vi "Send Receive.vi"(0 "Arduino Resource":T1={"VISA resource"="", "Board Type"=enum."Uno", "Connection Type"=enum."USB / Serial", "Bytes Per Packet (15)"=15}, 1 "Max Retries  (10)":i32=10, 5 "Data":u8[](array[numeric]), 7 "Bytes To Read (0)":u8, 9 "Time Out (100 ms)":i32=100, 11 "error in":errorcluster) -> (4 "Arduino Resource":T1={"VISA resource"="", "Board Type"=enum."Uno", "Connection Type"=enum."USB / Serial", "Bytes Per Packet (15)"=15}, 8 "Read Buffer":string, 15 "error out":errorcluster)   [LabVIEW 2015, in "LabVIEW Interface for Arduino.lvlib"]
uses:
  <vilib>/LabVIEW Interface for Arduino/LabVIEW Interface for Arduino.lvlib
  <vilib>/LabVIEW Interface for Arduino/Type Defs/Arduino Resource.ctl
  <vilib>/LabVIEW Interface for Arduino/Type Defs/Board Type.ctl
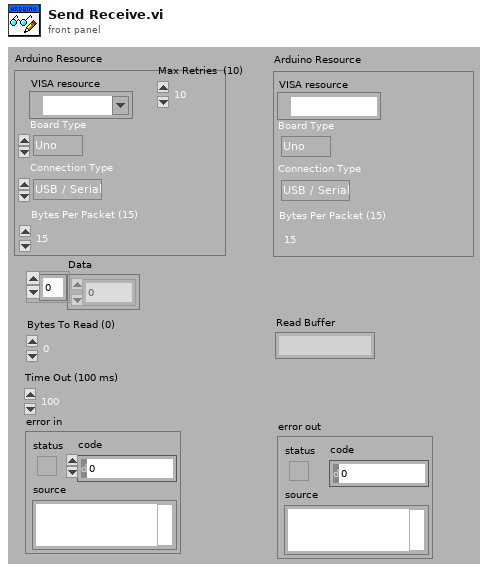
[diagram p1: front panel]
types:
  T1 = typedef "LabVIEW Interface for Arduino.lvlib/Arduino Resource.ctl" = cluster{"VISA resource":refnum<visa-resource-name>, "Board Type":T2, "Connection Type":enum8{"USB / Serial"}, "Bytes Per Packet (15)":u8}
  T2 = typedef "LabVIEW Interface for Arduino.lvlib/Board Type.ctl" = enum16{"Uno", "Dimuelanove w/Atmega 328", "Mega 2560"}
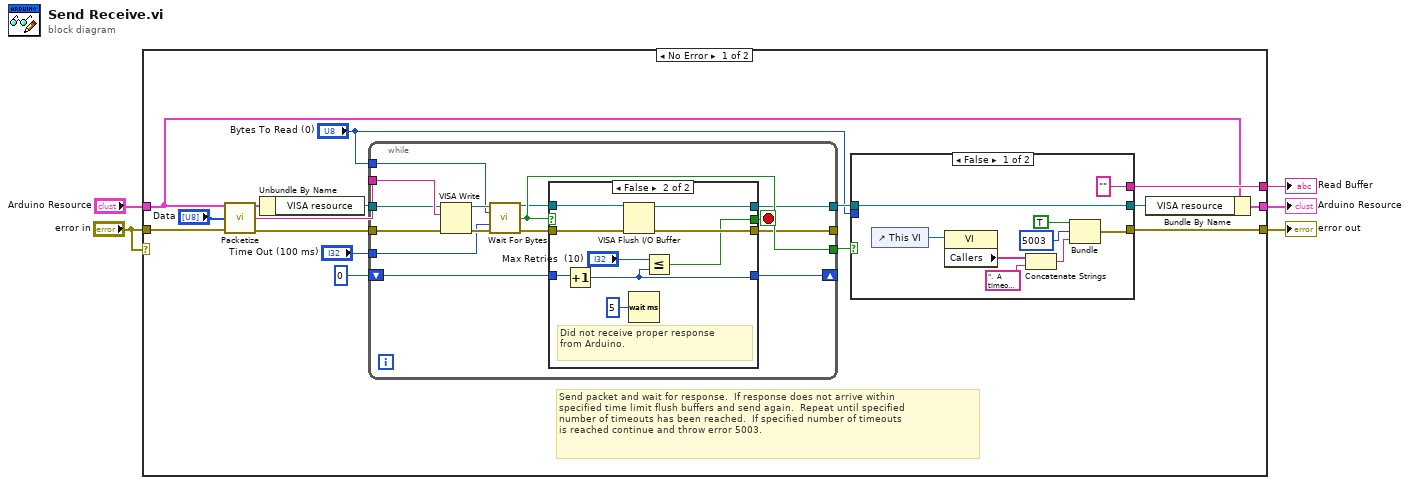
[diagram p0: block diagram]
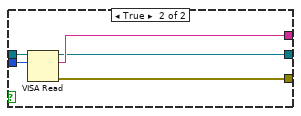
[diagram p3: hidden frame]
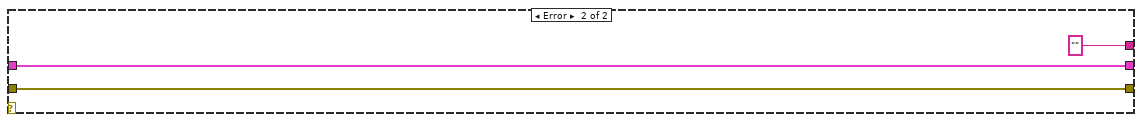
[diagram p4: hidden frame]
diagram:
  n1 = case shown="No Error" "error in" {
    tunnel: [w21 w65] -> w5
    tunnel: [w18 "" ("read buffer")] -> w4
    tunnel: "error in" -> [w6 w65]
    tunnel: "Arduino Resource" -> [w8 w66]
    tunnel: [w14 w66] -> w2
    frame No Error {
      # "Send packet and wait for response.  If response does not arrive within \nspecified time limit flush buffers and send again.  Repeat until specified \nnumber of timeouts has been reached.  If specified number of timeouts\nis reached continue and throw error 5003."
      n2 = call <vilib>:"Packetize.vi"("Arduino Resource"=w8, "Data"="Data", "error in"=w6) -> ("Arduino Resource"=w9:T1, "Packet"=w19:string, "error out"=w7:errorcluster)  [unwired: 10 in]
      n3 = Unbundle By Name(w9) -> ("VISA resource"=w16:refnum<visa-resource-name>)
      n4 = while {
        tunnel: w19 -> [w36]
        tunnel: [w24] -> w17
        tunnel: w7 -> [w33]
        tunnel: w16 -> [w32]
        tunnel: "Bytes To Read (0)" -> [w31]
        tunnel: "Time Out (100 ms)" -> [w30]
        tunnel: [w26] -> w11
        shift-right: [w28] -> _
        shift-left: 0 -> [w29]
        tunnel: [w22] -> _
        stop <- w27 stop-if-true
        n5 = VISA Write(VISA resource name=w32, write buffer=w36, error in (no error)=w33) -> (VISA resource name out=w34:refnum<visa-resource-name>, error out=w35:errorcluster)  [unwired: 1 out]
        n6 = call <vilib>:"Wait For Bytes.vi"("VISA resource"=w34, "Bytes To Read"=w31, "Time Out (100 ms)"=w30, "error in"=w35) -> ("VISA resource"=w23:refnum<visa-resource-name>, "Bytes Available?"=w26:bool, "error out"=w25:errorcluster)  [unwired: 9 in]
        n7 = case shown="False" w26 {
          selector: w26 -> [w39 _]
          tunnel: w29 -> [w40 w49]
          tunnel: [w40 w42] -> w28
          tunnel: [w39 w41] -> w27
          tunnel: w25 -> [w37 w47]
          tunnel: [w38 w46] -> w24
          tunnel: w23 -> [w38 w45]
          tunnel: [w37 w44] -> w22
          frame True {
          }
          frame False {
            # "Did not receive proper response\nfrom Arduino."
            n8 = Increment(x=w49) -> (x+1=w42:i32)
            n9 = VISA Flush I/O Buffer(VISA resource name=w45, error in (no error)=w47) -> (VISA resource name out=w46:refnum<visa-resource-name>, error out=w44:errorcluster)  [unwired: 1 in]
            n10 = Wait (ms)(milliseconds to wait=u32 5) -> ()  [unwired: 1 out]
            n11 = Less Or Equal?(x="Max Retries  (10)", y=w42) -> (x <= y?=w41:bool)
          }
        }
      }
      n12 = case shown="False" w11 {
        tunnel: [w53 w63] -> w21
        tunnel: ["" ("read buffer") w62] -> w18
        tunnel: w17 -> [w58 w61]
        tunnel: [w58 w60] -> w15
        tunnel: "Bytes To Read (0)" -> [_ w59]
        frame False {
          n13 = control-ref of="This VI"() -> (w54:refnum<vi>)
          n14 = property class="VI"(reference=w54) -> ("Callers"=w55:string[])  [unwired: 1 in, 2 out]
          n15 = Concatenate Strings(w55, ".  A timeout occurred while trying to read form the Arduino." ("string")) -> (w52:string)
          n16 = Bundle(TRUE, "code"=5003, w52) -> (w53:cluster{bool, "code":i32, string})  [unwired: 1 in]
        }
        frame True {
          n17 = VISA Read(VISA resource name=w61, byte count=w59) -> (VISA resource name out=w60:refnum<visa-resource-name>, read buffer=w62:string, error out=w63:errorcluster)  [unwired: 1 in, 1 out]
        }
      }
      n18 = Bundle By Name(cluster=w8, "VISA resource"=w15) -> (w14:T1)
    }
    frame Error {
    }
  }
  "error out" <- w5
  "Read Buffer" <- w4
  "Arduino Resource" <- w2
